vi "Test Compare Without Description.vi"(8 "error in (no error)":errorcluster, 11 "Test Test Case in":refnum<class "Test Test Case.lvclass">) -> (0 "error out":errorcluster, 3 "Test Test Case out":refnum<class "Test Test Case.lvclass">)   [LabVIEW 2020, in "Test Test Case.lvclass"]
uses:
  Test Test Case.lvclass
  C:/Git/astemes-lunit/source/Framework/Test Case/LUnit Test Case.lvclass
  source/Framework/Test Case/LUnit Test Case.lvclass/LUnit Test Case.ctl
  47fd1b1a-52c1-4c97-955d-790956f025ad.vi
  source/Framework/Test Case/Assertions/Pass.vi
  source/Framework/Test Case/Assertions/Fail.vi
  source/Framework/Test Case/Private/SubVIs/Compare Variants.vi
  source/Framework/Test Case/Private/SubVIs/Describe Comparison.vi
  source/Framework/Test Case/Private/SubVIs/Set Assertion Type.vi
  source/Framework/Test Case/Private/SubVIs/Add test result.vi
  source/Framework/Test Case/Private/SubVIs/Variant to string.vi
  source/Framework/Result Types/Case Result/Public/Record Assertion Result.vi
  source/Framework/Result Types/Method Result/Public/Aggregate Assertion Results.vi
  source/Framework/Result Types/Method Result/Private/Merge Status.vi
  source/Framework/Result Types/Method Result/Private/Concatenate result strings.vi
  <vilib>/Utility/Data Type/Get Type Information.vi
  <vilib>/Utility/LVClass/Get LV Class Name.vi
  Test Test Case.lvclass/Test Test Case.ctl
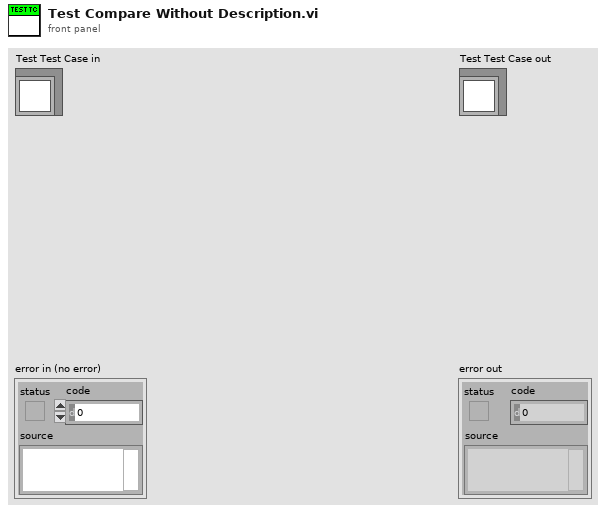
[diagram p1: front panel]
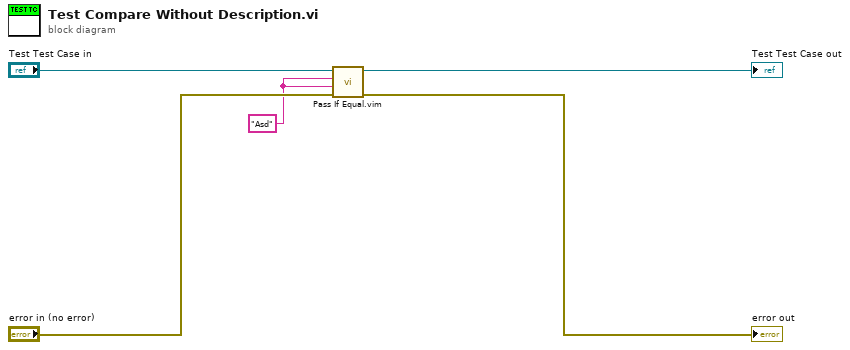
[diagram p0: block diagram]
diagram:
  w1 = "Asd"
  n1 = call "Pass If Equal.vim"("error in (no error)"="error in (no error)", "Actual"=w1, "Expected"=w1, "LUnit Test Case In"="Test Test Case in") -> ("error out"=→"error out":errorcluster, "LUnit Test Case Out"=→"Test Test Case out":refnum<class "Test Test Case.lvclass">)  [unwired: 6 in]
